vi "Read NumberOfRobots.vi"(8 "error in (no error)":errorcluster, 11 "DeadBallPlayVSS in":refnum<class "DeadBallPlayVSS.lvclass">) -> (0 "error out":errorcluster, 2 "NumberOfRobots":dbl, 3 "DeadBallPlayVSS out":refnum<class "DeadBallPlayVSS.lvclass">)   [LabVIEW 2023, in "DeadBallPlayVSS.lvclass"]
uses:
  DeadBallPlayVSS.lvclass
  DeadBallPlayVSS.lvclass/DeadBallPlayVSS.ctl
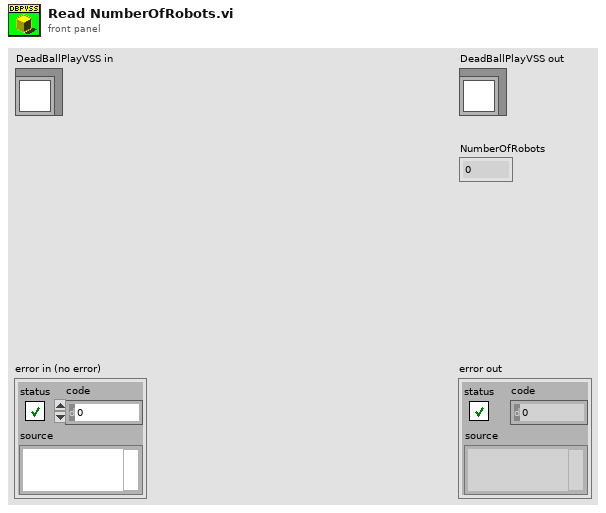
[diagram p1: front panel]
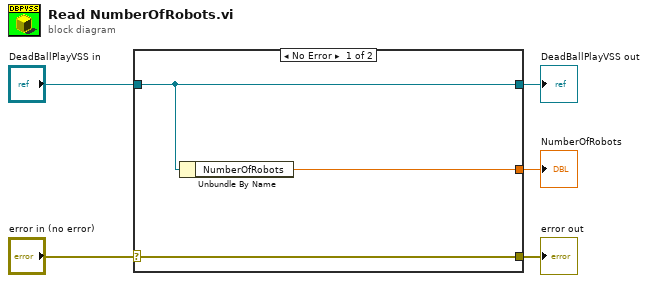
[diagram p0: block diagram]
diagram:
  n1 = case shown="No Error" "error in (no error)" {
    selector: "error in (no error)" -> [w8 w9]
    tunnel: [w8 w9] -> w4
    tunnel: [w7 w10] -> w2
    tunnel: "DeadBallPlayVSS in" -> [w7 w10]
    tunnel: [w6 _] -> w1
    frame No Error {
      n2 = Unbundle By Name(w7) -> ("NumberOfRobots"=w6:dbl)
    }
    frame Error {
    }
  }
  "error out" <- w4
  "DeadBallPlayVSS out" <- w2
  "NumberOfRobots" <- w1
